vi "PH_GUI.set waveform graph GUI object.vi"(2 "Graph GUI Ref":refnum<vi>, 3 "Values":dbl[](array[numeric]), 5 "error in":errorcluster) -> (19 "error out":errorcluster)   [LabVIEW 2014, in "PH_Common.lvlib"]
doc: "Sets value and more for the referenced GUI object."
uses:
  PH_Common.lvlib
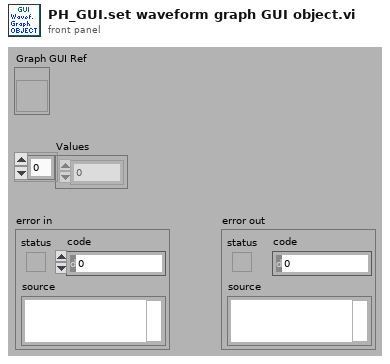
[diagram p1: front panel]
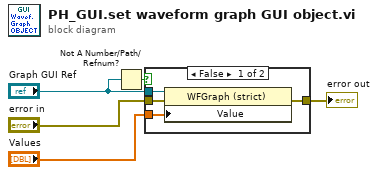
[diagram p0: block diagram]
diagram:
  n1 = Not A Number/Path/Refnum?(number/path/refnum="Graph GUI Ref") -> (NaN/Path/Refnum?=w4:bool)
  n2 = case shown="False" w4 {
    tunnel: "Graph GUI Ref" -> [w9 _]
    tunnel: "Values" -> [w8 _]
    tunnel: "error in" -> [w7 w10]
    tunnel: [w6 w10] -> w3
    frame False {
      n3 = property class="WFGraph (strict)"(reference=w9, error in=w7, "Value"=w8) -> (error out=w6:errorcluster)  [unwired: 1 out]
    }
    frame True {
    }
  }
  "error out" <- w3
